vi "appendXMLReference.vi"(8 "error in (no error)":errorcluster, 9 "Reference Path":path, 10 "Parent Camera Node":refnum<k20>, 11 "DOM document in":refnum<k20>) -> (0 "error out":errorcluster)   [LabVIEW 2013]
uses:
  <resource>/objmgr/DOMUserDefRef.rc
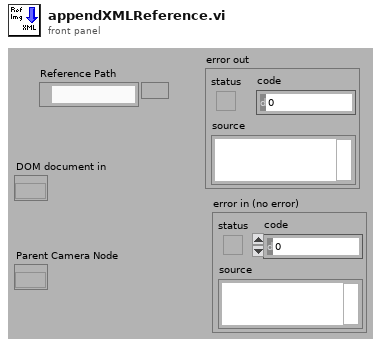
[diagram p1: front panel]
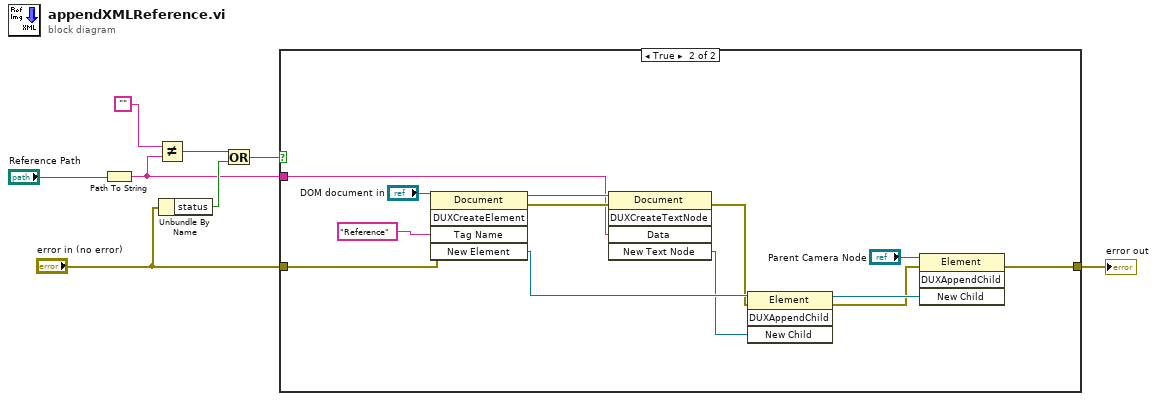
[diagram p0: block diagram]
diagram:
  n1 = Path To String(path="Reference Path") -> (string=w1:string)
  n2 = Not Equal?(x="", y=w1) -> (x != y?=w5:bool)
  n3 = Unbundle By Name("error in (no error)") -> ("status"=w4:bool)
  n4 = Or(x=w5, y=w4) -> (x .or. y?=w2:bool)
  n5 = case shown="True" w2 {
    tunnel: "error in (no error)" -> [w9 w15]
    tunnel: [w9 w11] -> w7
    tunnel: w1 -> [_ w10]
    frame False {
    }
    frame True {
      n6 = invoke class="Document" method="DUXCreateElement"(reference="DOM document in", error in=w15, "Tag Name"="Reference") -> (reference out=w21:refnum<k20>, error out=w14:errorcluster, "New Element"=w19:refnum<k20>)  [unwired: 2 in, 2 out]
      n7 = invoke class="Document" method="DUXCreateTextNode"(reference=w21, error in=w14, "Data"=w10) -> (error out=w13:errorcluster, "New Text Node"=w18:refnum<k20>)  [unwired: 2 in, 3 out]
      n8 = invoke class="Element" method="DUXAppendChild"(reference=w19, error in=w13, "New Child"=w18) -> (reference out=w16:refnum<k20>, error out=w12:errorcluster)  [unwired: 1 in, 2 out]
      n9 = invoke class="Element" method="DUXAppendChild"(reference="Parent Camera Node", error in=w12, "New Child"=w16) -> (error out=w11:errorcluster)  [unwired: 1 in, 3 out]
    }
  }
  "error out" <- w7
